vi "Recursive file name search.vi"(6 "Use Extensions (T)":bool=TRUE, 8 "error in":errorcluster, 10 "File Name":string, 11 "Top Level Dir":path) -> (0 "error out":errorcluster, 2 "Found?":bool, 3 "Path":path)   [LabVIEW 2013, in "FileIO lib.lvlib"]
uses:
  FileIO lib.lvlib
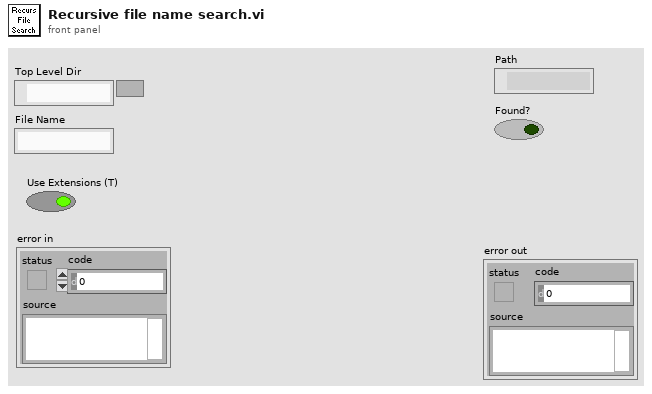
[diagram p1: front panel]
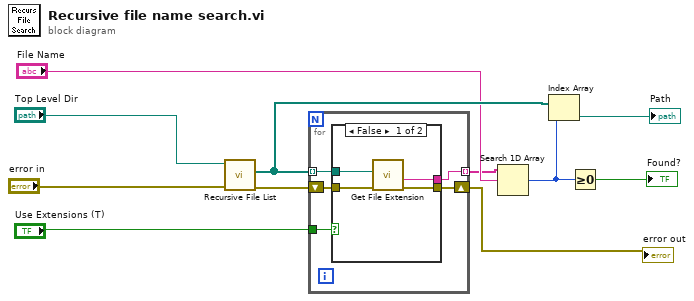
[diagram p0: block diagram]
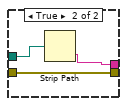
[diagram p2: hidden frame]
diagram:
  n1 = call <vilib>:"Recursive File List.vi"("error in (no error)"="error in", "Folder Path"="Top Level Dir") -> ("error out"=w3:errorcluster, "All Files in Dir"=w8:path[])  [unwired: 1 in, 7 out]
  n2 = for {
    tunnel: w8 -> [w16] mode=indexing
    tunnel: [w15] -> w6 mode=indexing
    shift-right: [w13] -> w2
    shift-left: w3 -> [w14]
    tunnel: "Use Extensions (T)" -> [w12]
    n3 = case shown="False" w12 {
      tunnel: w16 -> [w20 w22]
      tunnel: [w19 w21] -> w15
      tunnel: w14 -> [w18 w23]
      tunnel: [w17 w23] -> w13
      frame False {
        n4 = call <vilib>:"Get File Extension.vi"("error in (no error)"=w18, "file"=w20) -> ("error out"=w17:errorcluster, "filename without extension"=w19:string)  [unwired: 8 out]
      }
      frame True {
        n5 = Strip Path(path=w22) -> (name=w21:string)  [unwired: 1 out]
      }
    }
  }
  "error out" <- w2
  n6 = Search 1D Array(1D array=w6, element="File Name") -> (index of element=w9:i32)  [unwired: 1 out]
  n7 = Index Array(array=w8, index=w9) -> (element=→"Path":path)
  n8 = Greater Or Equal To 0?(x=w9) -> (x >= 0?=→"Found?":bool)
